vi "test2_device.vi"() -> ()   [LabVIEW 2017]
panel:
  out "数字 2":i32
  out "数字":i32
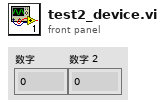
[diagram p1: front panel]
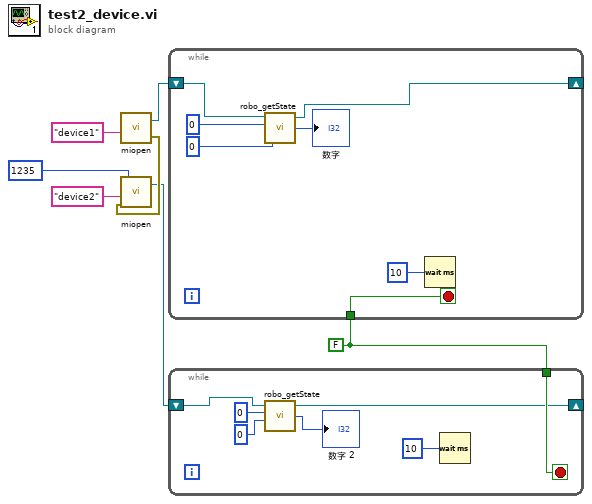
[diagram p0: block diagram]
diagram:
  w2 = FALSE
  n1 = call "miopen.vi"("name"="device1") -> ("错误输出"=w5:errorcluster, "VISA资源名称输出"=w3:refnum<visa-resource-name>)  [unwired: 3 in]
  n2 = call "miopen.vi"("错误输入（无错误）"=w5, "name"="device2", "port"=u16 1235) -> ("VISA资源名称输出"=w1:refnum<visa-resource-name>)  [unwired: 1 in, 1 out]
  n3 = while {
    shift-right: [w11] -> _
    shift-left: w3 -> [w9]
    tunnel: w2 -> [w8]
    stop <- w8 stop-if-true
    n4 = call "robo_getState.vi"("输入 2"=0, "输入 1"=0, "VISA资源名称"=w9) -> ("数字"=→"数字":i32, "VISA资源名称输出"=w11:refnum<visa-resource-name>)  [unwired: 1 in, 1 out]
    n5 = Wait (ms)(milliseconds to wait=u32 10 ("等待时间（毫秒）")) -> ()  [unwired: 1 out]
  }
  n6 = while {
    tunnel: w2 -> [w21]
    shift-right: [w17] -> _
    shift-left: w1 -> [w16]
    stop <- w21 stop-if-true
    n7 = call "robo_getState.vi"("输入 2"=0, "输入 1"=0, "VISA资源名称"=w16) -> ("数字"=→"数字 2":i32, "VISA资源名称输出"=w17:refnum<visa-resource-name>)  [unwired: 1 in, 1 out]
    n8 = Wait (ms)(milliseconds to wait=u32 10 ("等待时间（毫秒）")) -> ()  [unwired: 1 out]
  }
